vi "Set IPS PSU Targets.vi"(8 "error in (no error)":errorcluster, 9 "Target Field Rate (T/min)":dbl format="%#.2f", 10 "Target Field (T)":dbl format="%#.2f", 11 "Instrument.Oxford1820 in":refnum<class "Instrument.Oxford1820.lvclass">) -> (0 "error out":errorcluster, 2 "Response":string, 3 "Instrument.Oxford1820 out":refnum<class "Instrument.Oxford1820.lvclass">)   [LabVIEW 2016, in "Instrument.Oxford1820.lvclass"]
uses:
  Instrument.Oxford1820.lvclass
  Instrument.Oxford1820.lvclass/Instrument.Oxford1820.ctl
  <instrlib>/Mercury iXX/Public/Libraries/Magnet/Open/Open Magnet Device.vi
  <instrlib>/Mercury iXX/Public/Libraries/Magnet/Signals/Set/Target Field Rate (Set).vi
  <instrlib>/Mercury iXX/Public/Libraries/Magnet/Signals/Set/Target Field (Set).vi
  <instrlib>/Mercury iXX/Mercury iXX.lvlib
  <instrlib>/Mercury iXX/Public/Libraries/Magnet.lvlib
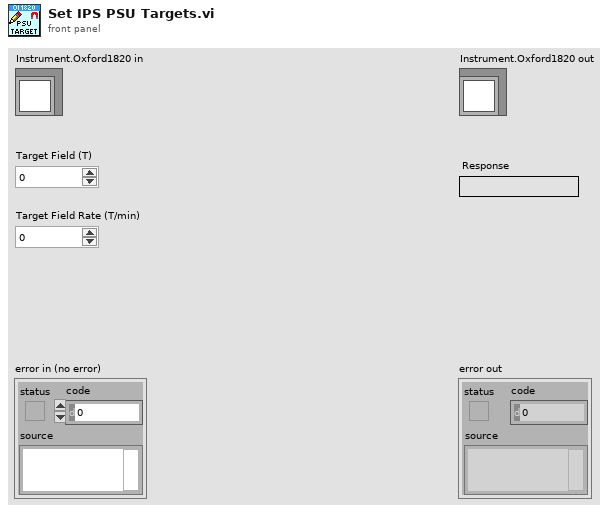
[diagram p1: front panel]
types:
  T1 = typedef "Mercury iXX.lvlib/Mercury Reference.ctl" = cluster{"Comms":refnum<visa-resource-name>, "Device ID":string[], "Comms Layer":T2, "Command":string, "Query reference":T3}
  T2 = typedef "Mercury iXX.lvlib/Comms Transport Layer.ctl" = enum16{"Ethernet TCP/IP", "USB", "ISOBus - RS-232", "GPIB"}
  T3 = typedef "Mercury iXX.lvlib/Query Dynamic Reference.ctl" = refnum<vi>
  T4 = typedef "Mercury iXX.lvlib/Response String.ctl" = string
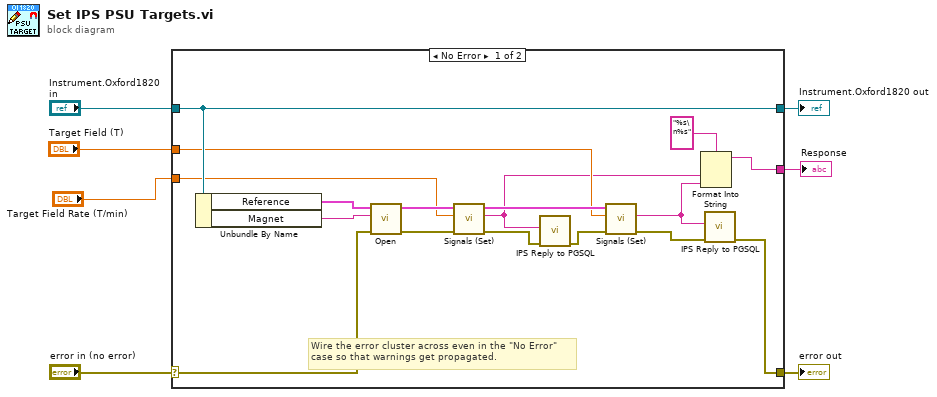
[diagram p0: block diagram]
diagram:
  n1 = case shown="No Error" "error in (no error)" {
    selector: "error in (no error)" -> [w21 w26]
    tunnel: [w12 w26] -> w6
    tunnel: [w24 w25] -> w4
    tunnel: "Instrument.Oxford1820 in" -> [w24 w25]
    tunnel: [w8 _] -> w3
    tunnel: "Target Field (T)" -> [w14 _]
    tunnel: "Target Field Rate (T/min)" -> [w13 _]
    frame No Error {
      # "Wire the error cluster across even in the \"No Error\"\ncase so that warnings get propagated."
      n2 = Unbundle By Name(w24) -> ("Reference"=w22:T1, "Magnet"=w23:string)
      n3 = call-poly <instrlib>:"Open.vi"("error in (no error)"=w21, "Device Identifier"=w23, "Mercury Reference In"=w22) -> ("error out"=w15:errorcluster, "Mercury Reference Out"=w16:T1)  [unwired: 7 out]
      n4 = call-poly <instrlib>:"Signals (Set).vi"("error in"=w15, "Target Field Rate"=w13, "Mercury Reference In"=w16) -> ("error out"=w19:errorcluster, "Response"=w9:T4, "Mercury Reference Out"=w17:T1)  [unwired: 2 in, 4 out]
      n5 = call "IPS Reply to PGSQL.vi"("error in (no error)"=w19, "Response"=w9) -> ("error out"=w18:errorcluster)  [unwired: 9 in]
      n6 = call-poly <instrlib>:"Signals (Set).vi"("error in"=w18, "Target Field"=w14, "Mercury Reference In"=w17) -> ("error out"=w20:errorcluster, "Response"=w10:T4)  [unwired: 2 in, 5 out]
      n7 = Format Into String(format string="%s\n%s", w9, w10) -> (resulting string=w8:string)  [unwired: 2 in, 1 out]
      n8 = call "IPS Reply to PGSQL.vi"("error in (no error)"=w20, "Response"=w10) -> ("error out"=w12:errorcluster)  [unwired: 9 in]
    }
    frame Error {
    }
  }
  "error out" <- w6
  "Instrument.Oxford1820 out" <- w4
  "Response" <- w3
